vi "TCP - Open Connection.vi"(8 "error in (no error)":errorcluster, 11 "DAQ IP Address":string="192.168.1.1") -> (0 "error out":errorcluster, 3 "TCP Network Connection out":refnum<k5>)   [LabVIEW 2020]
doc: "Open a TCP connection to the DAQ"
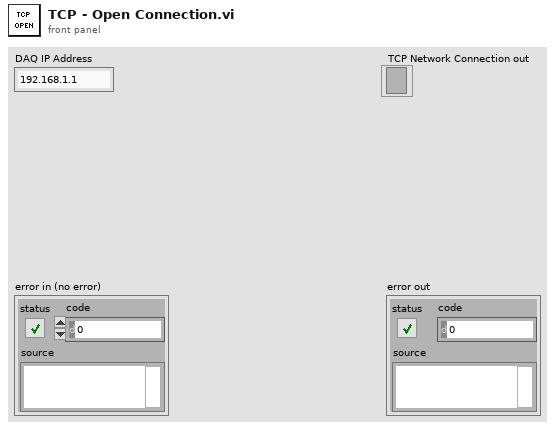
[diagram p1: front panel]
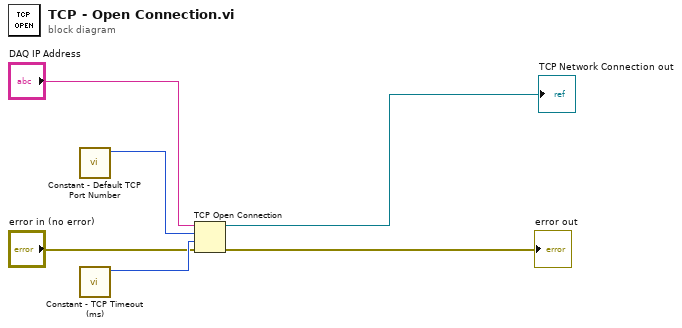
[diagram p0: block diagram]
diagram:
  n1 = call "Constant - Default TCP Port Number.vi"() -> ("Port"=w2:u16)  [unwired: 11 in]
  n2 = call "Constant - TCP Timeout (ms).vi"() -> ("timeout (ms)"=w6:i32)  [unwired: 11 in]
  n3 = TCP Open Connection(address="DAQ IP Address", remote port or service name=w2, timeout ms (60000)=w6, error in (no error)="error in (no error)") -> (connection ID=→"TCP Network Connection out":refnum<k5>, error out=→"error out":errorcluster)  [unwired: 1 in]
